vi "SetValue.vi"(6 "Replace?":bool, 8 "error in (no error)":errorcluster, 9 "Key":variant, 10 "Value":variant, 11 "Map in":refnum<class "Map.lvclass">) -> (0 "error out":errorcluster, 1 "Created New?":bool, 2 "Value":variant, 3 "Map out":refnum<class "Map.lvclass">)   [LabVIEW 2016, in "Map.lvclass"]
uses:
  <userlib>/836-libraries/Data_Structures/Map/Map.lvclass
  <userlib>/836-libraries/Data_Structures/Map/Map.lvclass/Map.ctl
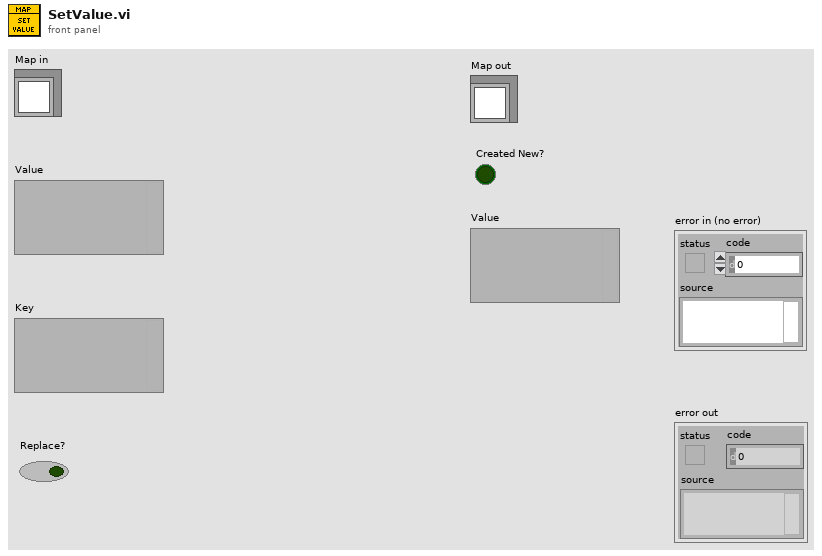
[diagram p1: front panel]
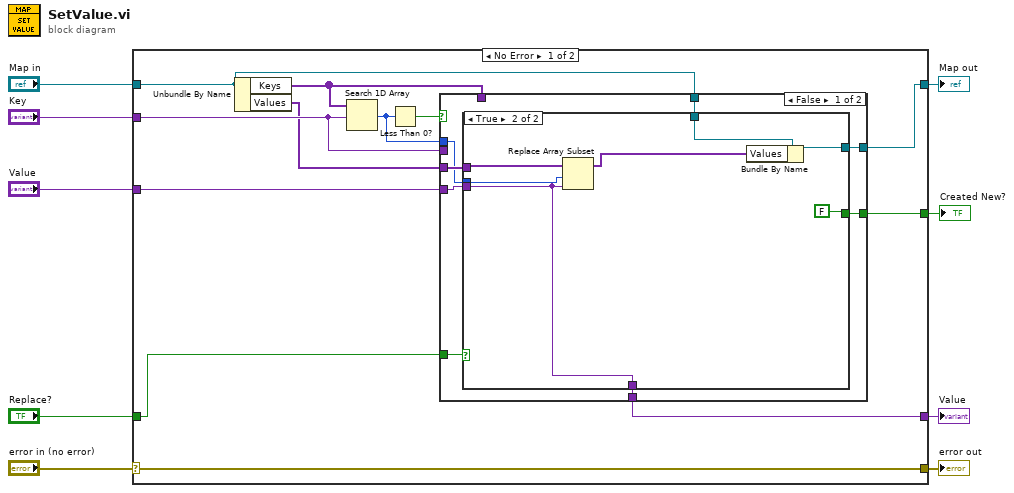
[diagram p0: block diagram]
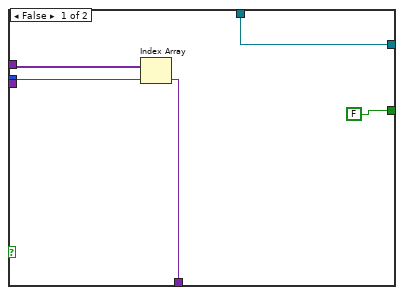
[diagram p2: hidden frame]
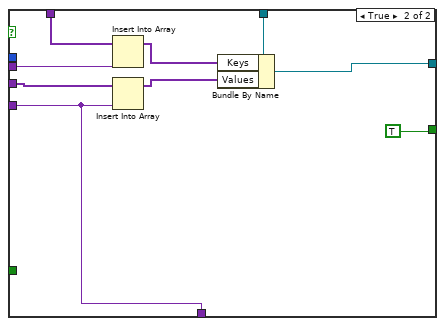
[diagram p3: hidden frame]
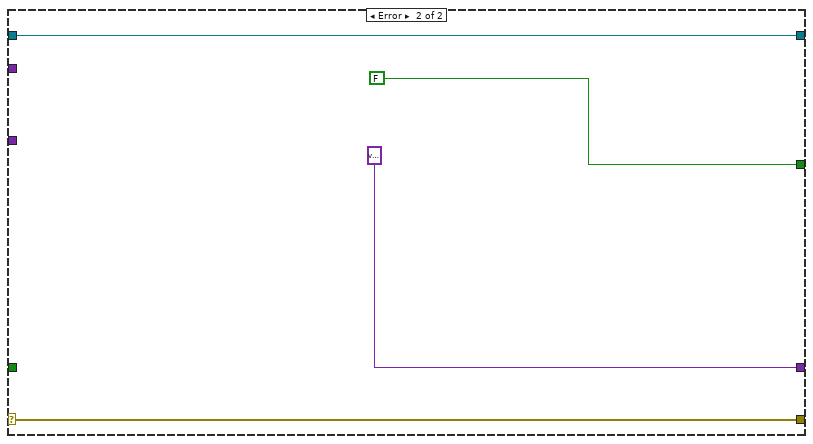
[diagram p4: hidden frame]
diagram:
  n1 = case shown="No Error" "error in (no error)" {
    selector: "error in (no error)" -> [w21 w53]
    tunnel: [w21 w53] -> w8
    tunnel: [w16 w54] -> w6
    tunnel: "Map in" -> [w19 w54]
    tunnel: "Key" -> [w14 _]
    tunnel: "Value" -> [w18 _]
    tunnel: "Replace?" -> [w12 _]
    tunnel: [w11 variant ("Value")] -> w2
    tunnel: [w10 FALSE ("Created New?")] -> w1
    frame No Error {
      n2 = Unbundle By Name(w19) -> ("Keys"=w15:variant[], "Values"=w13:variant[])
      n3 = Search 1D Array(1D array=w15, element=w14) -> (index of element=w17:i32)  [unwired: 1 in]
      n4 = Less Than 0?(x=w17) -> (x < 0?=w20:bool)
      n5 = case shown="False" w20 {
        tunnel: w19 -> [w26 w50]
        tunnel: w15 -> [_ w48]
        tunnel: w18 -> [w23 w43]
        tunnel: w17 -> [w27 _]
        tunnel: [w25 w49] -> w16
        tunnel: w14 -> [_ w47]
        tunnel: w13 -> [w28 w45]
        tunnel: w12 -> [w29 _]
        tunnel: [w24 w43] -> w11
        tunnel: [w22 TRUE] -> w10
        frame False {
          n6 = case shown="True" w29 {
            tunnel: w28 -> [w34 w41]
            tunnel: w27 -> [w33 w40]
            tunnel: w26 -> [w32 w38]
            tunnel: [w32 w39] -> w25
            tunnel: [w31 w36] -> w24
            tunnel: w23 -> [_ w36]
            tunnel: [FALSE FALSE] -> w22
            frame False {
              n7 = Index Array(array=w34, index=w33) -> (element=w31:variant)
            }
            frame True {
              n8 = Replace Array Subset(array=w41, new element=w36, index=w40) -> (w37:variant[])
              n9 = Bundle By Name(cluster=w38, "Values"=w37) -> (w39:refnum<class "Map.lvclass">)
            }
          }
        }
        frame True {
          n10 = Insert Into Array(array=w48, new element=w47) -> (w46:variant[])  [unwired: 1 in]
          n11 = Insert Into Array(array=w45, new element=w43) -> (w44:variant[])  [unwired: 1 in]
          n12 = Bundle By Name(cluster=w50, "Keys"=w46, "Values"=w44) -> (w49:refnum<class "Map.lvclass">)
        }
      }
    }
    frame Error {
    }
  }
  "error out" <- w8
  "Map out" <- w6
  "Value" <- w2
  "Created New?" <- w1
